vi "up_down_counter.vi"(1 "reset":bool, 2 "up":bool, 3 "down":bool) -> (0 "Value":i16)   [LabVIEW 2018]
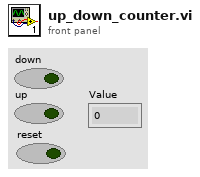
[diagram p1: front panel]
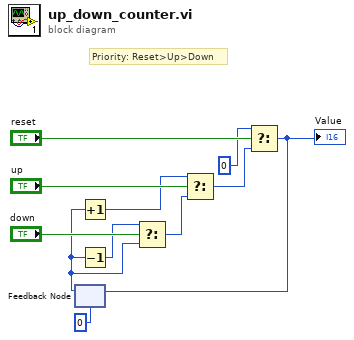
[diagram p0: block diagram]
diagram:
  # "Priority: Reset>Up>Down"
  n1 = feedback #1(i16 0) -> (w1:i16)
  n2 = Increment(x=w1) -> (x+1=w7:i16)
  n3 = Decrement(x=w1) -> (x-1=w3:i16)
  n4 = Select(t=w3, s="down", f=w1) -> (s? t:f=w8:i16)
  n5 = Select(t=w7, s="up", f=w8) -> (s? t:f=w6:i16)
  n6 = Select(t=i16 0, s="reset", f=w6) -> (s? t:f=w2:i16)
  "Value" <- w2
  n7 = feedback-in #1(w2) -> ()
